vi "DELETE MEbyte array to u16.vi"() -> ()   [LabVIEW 2024]
panel:
  out "*(type *) &x 2":i16
  out "*(type *) &x":u8[](array[numeric])
  out "size(s)":i32
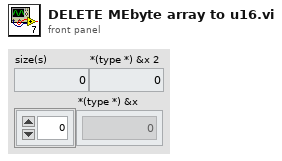
[diagram p1: front panel]
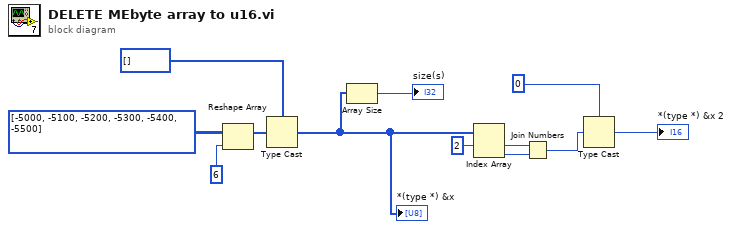
[diagram p0: block diagram]
diagram:
  n1 = Reshape Array(i16[][] [[-5000, -5100, -5200], [-5300, -5400, -5500]], 6 ("dimension size")) -> (w9:i16[])
  n2 = Type Cast(type=u8[] [], x=w9) -> (*(type *) &x=w7:u8[])
  "*(type *) &x" <- w7
  n3 = Array Size(array=w7) -> (size(s)=→"size(s)":i32)
  n4 = Index Array(array=w7, index #1=2 ("index")) -> (element #1=w3:u8, element #2=w2:u8)  [unwired: 1 in]
  n5 = Join Numbers(hi=w3, lo=w2) -> ((hi.lo)=w1:u16)
  n6 = Type Cast(type=i16 0, x=w1) -> (*(type *) &x=→"*(type *) &x 2":i16)
